vi "Close Ref.vi"(8 "Error In":errorcluster, 11 "DVR Ref":refnum<data-value>) -> (0 "Error Out":errorcluster)   [LabVIEW 2023, in "Arithemetic Operation.lvclass"]
doc: "The method accepts the DVR of class data as the input and closes the VI reference that the class holds."
uses:
  Arithemetic Operation.lvclass
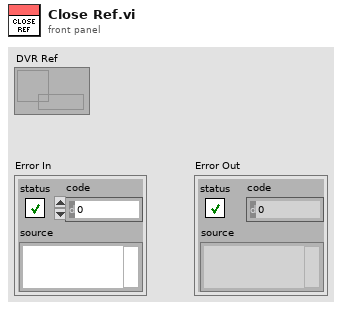
[diagram p1: front panel]
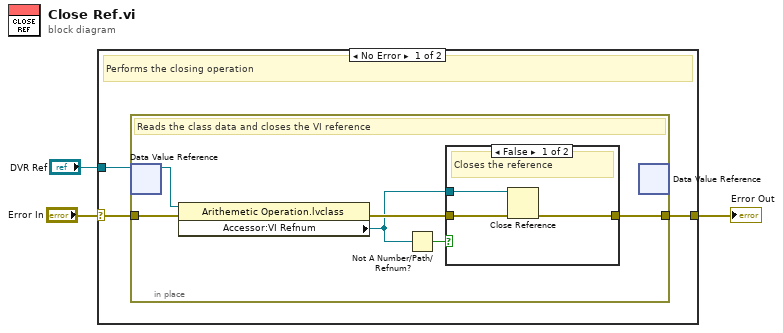
[diagram p0: block diagram]
diagram:
  n1 = case shown="No Error" "Error In" {
    selector: "Error In" -> [w5 w17]
    tunnel: "DVR Ref" -> [w4 _]
    tunnel: [w6 w17] -> w1
    frame No Error {
      # "Performs the closing operation"
      n2 = in-place {
        in-place-border: [w9] -> w6
        in-place-border: w5 -> [w8]
        # "Reads the class data and closes the VI reference"
        n3 = in-place-dvr #1(w4) -> (w7:refnum<class "Arithemetic Operation.lvclass">)  [unwired: 1 out]
        n4 = property class="Arithemetic Operation.lvclass"(reference=w7, error in=w8) -> (error out=w12:errorcluster, "Accessor:VI Refnum"=w10:refnum<vi>)  [unwired: 1 out]
        n5 = Not A Number/Path/Refnum?(number/path/refnum=w10) -> (NaN/Path/Refnum?=w11:bool)
        n6 = case shown="False" w11 {
          tunnel: w12 -> [w15 w16]
          tunnel: [w14 w16] -> w9
          tunnel: w10 -> [w13 _]
          frame False {
            # "Closes the reference"
            n7 = Close Reference(reference=w13, error in (no error)=w15) -> (error out=w14:errorcluster)
          }
          frame True {
          }
        }
        n8 = in-place-dvr #1() -> ()  [unwired: 1 in, 2 out]
      }
    }
    frame Error {
    }
  }
  "Error Out" <- w1
